vi "Dialog Preview Message.vi"(8 "error in (no error)":errorcluster) -> (0 "error out":errorcluster, 3 "Cancelled?":bool)   [LabVIEW 2012]
doc: "SciScan 1.2 160622"
panel:
  in  "Cancel Button":bool
  in  "OK Button":bool
  # "Preview will step through every macro command and ask you to confirm the settings.\nPreview will not execute any recording."
  # "WARNING: Preview will execute stage move commands (if any)\nPlease ensure that this will not cause any damage to your \nequipment or sample. If you are unsure, please press Cancel."
  # "Press OK to start preview.\nPress Cancel to abort."
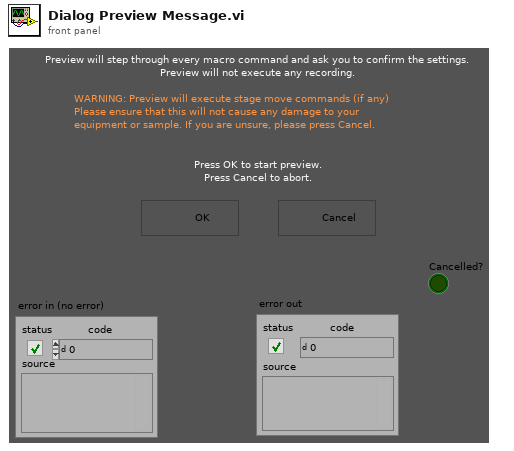
[diagram p1: front panel]
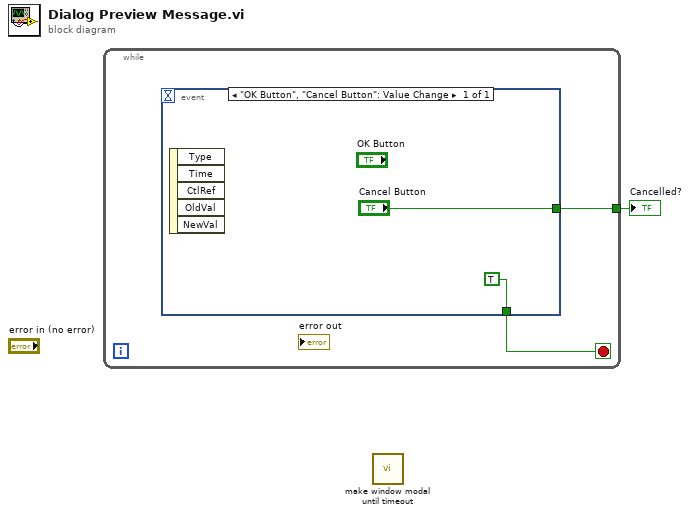
[diagram p0: block diagram]
diagram:
  n1 = while {
    tunnel: [w3] -> w1
    stop <- w2 stop-if-true
    n2 = event shown="[0] \"OK Button\", \"Cancel Button\": Value Change" {
      selector: _ -> [_]
      dyn-events: _ -> [_]
      timeout: _ -> [_]
      tunnel: ["Cancel Button"] -> w3
      tunnel: [TRUE] -> w2
      event "OK Button", "Cancel Button": Value Change {
        n3 = event-data() -> ()  [unwired: 1 in, 5 out]
      }
    }
  }
  "Cancelled?" <- w1
  n4 = call "make window modal until timeout.vi"() -> ()  [unwired: 12 in]
